vi "GetTeamData.vi"(10 "Team #":string) -> (0 "Pictures":string[](array[string]), 1 "Data":string, 2 "Location":string, 3 "Name":string)   [LabVIEW 2018]
uses:
  <vilib>/Utility/config.llb/Read Key (String).vi
  <vilib>/Utility/config.llb/NI_LVConfig.lvlib
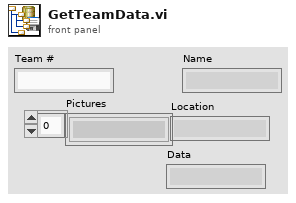
[diagram p1: front panel]
types:
  T1 = typedef "NI_LVConfig.lvlib/Config Data RefNum.ctl" = refnum<k1>
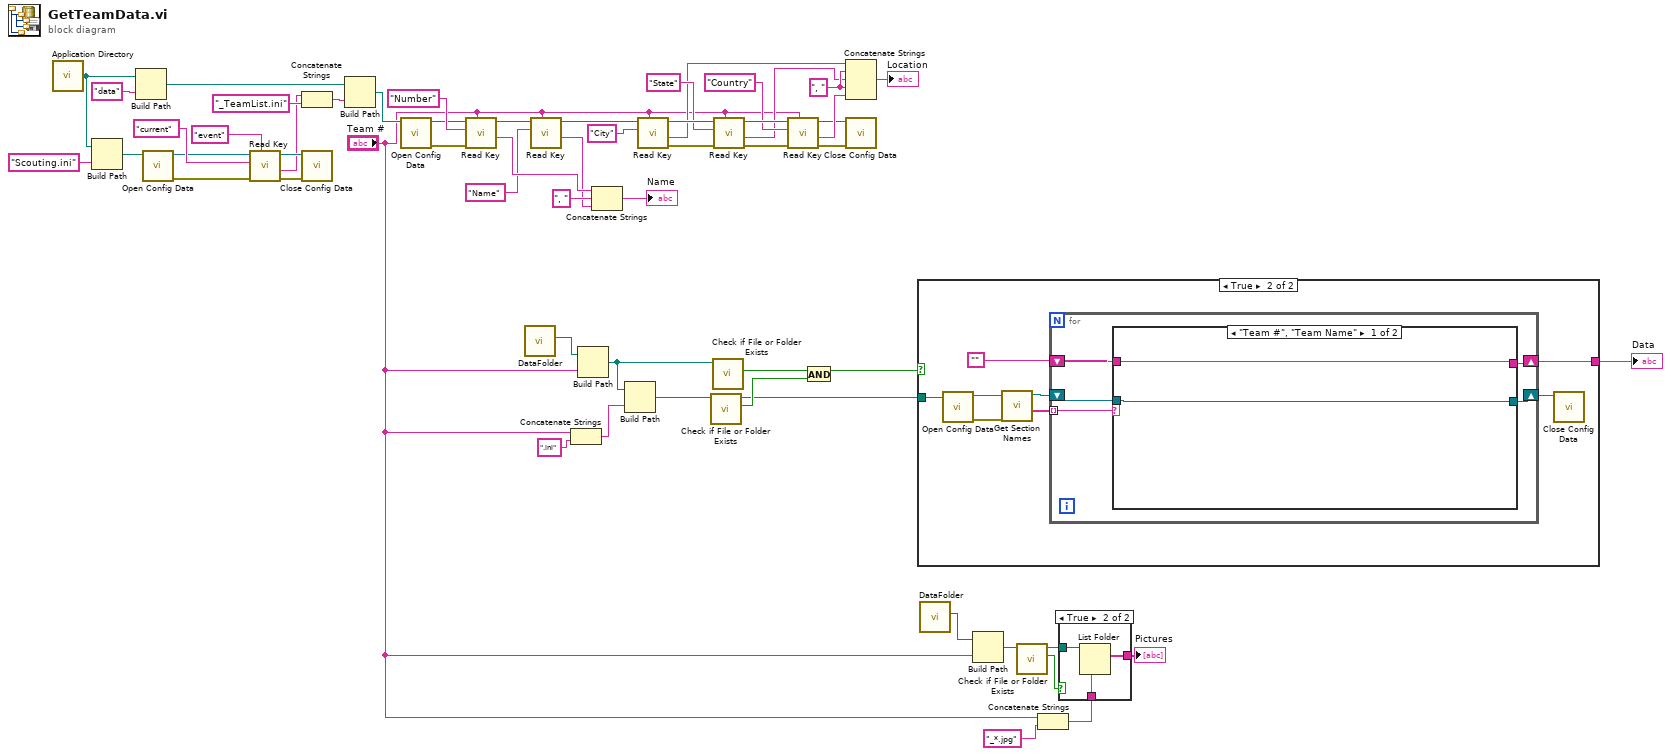
[diagram p0: block diagram]
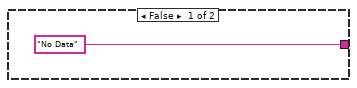
[diagram p3: hidden frame]
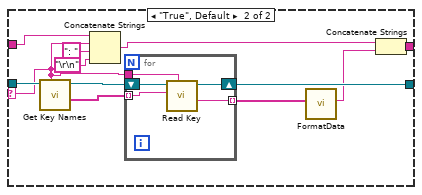
[diagram p4: hidden frame]
diagram:
  w25 = ", " ("string")
  n1 = call <vilib>:"Application Directory.vi"() -> ("Application Directory"=w46:path)
  n2 = Build Path(base path=w46, name or relative path="Scouting.ini") -> (appended path=w39:path)
  n3 = Build Path(base path=w46, name or relative path="data") -> (appended path=w41:path)
  n4 = call <vilib>:"Open Config Data.vi"("configuration file path"=w39) -> ("error out"=w33:errorcluster, "refnum"=w34:T1)  [unwired: 8 in, 1 out]
  n5 = call-poly <vilib>:"Read Key.vi"("section"="event" ("key"), "error in (no error)"=w33, "key"="current" ("section"), "refnum"=w34) -> ("error out"=w35:errorcluster, "value"=w26:string, "refnum out"=w36:T1)  [unwired: 4 in, 1 out]
  n6 = Concatenate Strings(w26, "_TeamList.ini" ("string")) -> (w42:string)
  n7 = call <vilib>:"Close Config Data.vi"("error in (no error)"=w35, "refnum"=w36) -> ()  [unwired: 8 in, 2 out]
  n8 = Build Path(base path=w41, name or relative path=w42) -> (appended path=w45:path)
  n9 = call <vilib>:"Open Config Data.vi"("configuration file path"=w45) -> ("error out"=w47:errorcluster, "refnum"=w48:T1)  [unwired: 8 in, 1 out]
  n10 = call-poly <vilib>:"Read Key.vi"("section"="Team #", "error in (no error)"=w47, "key"="Number", "refnum"=w48) -> ("value"=w53:string, "refnum out"=w50:T1)  [unwired: 4 in, 2 out]
  n11 = call "DataFolder.vi"() -> ("appended path"=w18:path)  [unwired: 11 in]
  n12 = call-poly <vilib>:"Read Key.vi"("section"="Team #", "key"="Name", "refnum"=w50) -> ("value"=w52:string, "refnum out"=w56:T1)  [unwired: 5 in, 2 out]
  n13 = Concatenate Strings("Team #", ".ini" ("format string")) -> (w15:string)
  n14 = Build Path(base path=w18, name or relative path="Team #") -> (appended path=w14:path)
  n15 = Concatenate Strings(w53, ", " ("string"), w52) -> (→"Name":string)
  n16 = Build Path(base path=w14, name or relative path=w15) -> (appended path=w13:path)
  n17 = call-poly <vilib>:"Read Key.vi"("section"="Team #", "key"="City", "refnum"=w56) -> ("error out"=w31:errorcluster, "value"=w24:string, "refnum out"=w32:T1)  [unwired: 5 in, 1 out]
  n18 = call <vilib>:"Check if File or Folder Exists.vi"("path"=w13) -> ("file or folder exists?"=w11:bool, "dup path"=w9:path)  [unwired: 8 in, 1 out]
  n19 = call <vilib>:"Check if File or Folder Exists.vi"("path"=w14) -> ("file or folder exists?"=w17:bool)  [unwired: 8 in, 2 out]
  n20 = call-poly <vilib>:"Read Key.vi"("section"="Team #", "error in (no error)"=w31, "key"="State", "refnum"=w32) -> ("error out"=w29:errorcluster, "value"=w23:string, "refnum out"=w30:T1)  [unwired: 4 in, 1 out]
  n21 = call-poly <vilib>:"Read Key.vi"("section"="Team #", "error in (no error)"=w29, "key"="Country", "refnum"=w30) -> ("error out"=w20:errorcluster, "value"=w22:string, "refnum out"=w19:T1)  [unwired: 4 in, 1 out]
  n22 = And(x=w17, y=w11) -> (x .and. y?=w12:bool)
  n23 = Concatenate Strings(w24, w25, w23, w25, w22) -> (→"Location":string)
  n24 = call <vilib>:"Close Config Data.vi"("error in (no error)"=w20, "refnum"=w19) -> ()  [unwired: 8 in, 2 out]
  n25 = case shown="True" w12 {
    tunnel: ["No Data" ("key") w59] -> w10
    tunnel: w9 -> [_ w66]
    frame False {
    }
    frame True {
      n26 = call <vilib>:"Open Config Data.vi"("configuration file path"=w66) -> ("error out"=w65:errorcluster, "refnum"=w64:T1)  [unwired: 8 in, 1 out]
      n27 = call <vilib>:"Get Section Names.vi"("error in (no error)"=w65, "refnum"=w64) -> ("section names"=w63:string[], "refnum out"=w62:T1)  [unwired: 7 in, 1 out]
      n28 = for {
        tunnel: w63 -> [w67] mode=indexing
        shift-right: [w69] -> w61
        shift-left: w62 -> [w71]
        shift-right: [w70] -> w59
        shift-left: "" -> [w68]
        n29 = case shown="\"Team #\", \"Team Name\"" w67 {
          selector: w67 -> [_ w76]
          tunnel: w71 -> [w72 w85]
          tunnel: [w73 w84] -> w70
          tunnel: [w72 w81] -> w69
          tunnel: w68 -> [w73 w80]
          frame "Team #", "Team Name" {
          }
          frame "True", Default {
            n30 = call <vilib>:"Get Key Names.vi"("section"=w76, "refnum"=w85) -> ("key names"=w83:string[], "refnum out"=w82:T1)  [unwired: 6 in, 2 out]
            n31 = Concatenate Strings(w80, w76, ": " ("string"), "\r\n") -> (w78:string)
            n32 = for {
              tunnel: w83 -> [w90] mode=indexing
              shift-right: [w88] -> w81
              shift-left: w82 -> [w89]
              tunnel: w76 -> [w87]
              tunnel: [w86] -> w75 mode=indexing
              n33 = call-poly <vilib>:"Read Key.vi"("section"=w87, "key"=w90, "refnum"=w89) -> ("value"=w86:string, "refnum out"=w88:T1)  [unwired: 5 in, 2 out]
            }
            n34 = call "FormatData.vi"("Array"=w75) -> ("data"=w74:string)  [unwired: 10 in]
            n35 = Concatenate Strings(w78, w74) -> (w84:string)
          }
        }
      }
      n36 = call <vilib>:"Close Config Data.vi"("refnum"=w61) -> ()  [unwired: 9 in, 2 out]
    }
  }
  "Data" <- w10
  n37 = call "DataFolder.vi"() -> ("appended path"=w8:path)  [unwired: 11 in]
  n38 = Build Path(base path=w8, name or relative path="Team #") -> (appended path=w7:path)
  n39 = call <vilib>:"Check if File or Folder Exists.vi"("path"=w7) -> ("file or folder exists?"=w1:bool, "dup path"=w4:path)  [unwired: 8 in, 1 out]
  n40 = Concatenate Strings("Team #", "_*.jpg" ("string")) -> (w5:string)
  n41 = case shown="True" w1 {
    tunnel: w5 -> [_ w93]
    tunnel: w4 -> [_ w92]
    tunnel: [_ w91] -> w3
    frame False {
    }
    frame True {
      n42 = List Folder(path=w92, pattern=w93) -> (filenames=w91:string[])  [unwired: 2 in, 3 out]
    }
  }
  "Pictures" <- w3
